vi "Purge Device List.vi"(8 "Error In":errorcluster, 11 "Device list":refnum<class "Device.lvclass">[](array[class])) -> (0 "Error Out":errorcluster, 3 "Device list out":refnum<class "Device.lvclass">[](array[class]))   [LabVIEW 2015]
uses:
  Device.lvclass
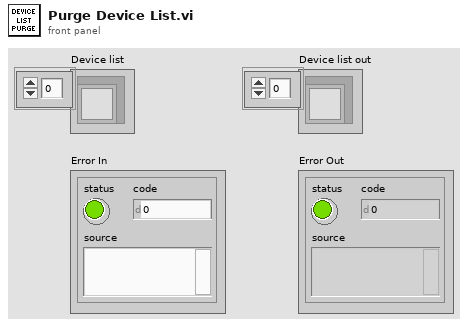
[diagram p1: front panel]
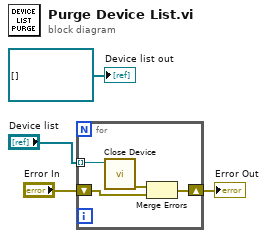
[diagram p0: block diagram]
diagram:
  n1 = for {
    tunnel: "Device list" -> [w8] mode=indexing
    shift-right: [w6] -> w2
    shift-left: "Error In" -> [w5]
    n2 = call "Close Device.vi"("Device"=w8) -> ("error out"=w7:errorcluster)  [unwired: 9 in, 1 out]
    n3 = Merge Errors(w7, w5) -> (w6:errorcluster)
  }
  "Error Out" <- w2
  "Device list out" <- refnum<class "Device.lvclass">[] [] ("Complete device list")
